vi "setSpectTempSetpoint.vi"(8 "error in (no error)":errorcluster, 9 "command_setSpectTempSetpoint":T1, 10 "model in":refnum<class "IModel.lvclass">, 11 "EnabledState in":refnum<class "EnabledState.lvclass">) -> (0 "error out":errorcluster, 2 "model out":refnum<class "IModel.lvclass">, 3 "EnabledState out":refnum<class "EnabledState.lvclass">)   [LabVIEW 2016, in "States.lvlib" / "EnabledState.lvclass"]
uses:
  EnabledState.lvclass
  IModel/IModel.lvclass
  ts_sallv_sedspectrometer/DataTypes/command_setSpectTempSetpoint.ctl
  DefaultState/DefaultState.lvclass
  ts_sallv_sedspectrometer/SALLV_sedSpectrometer.lvlib
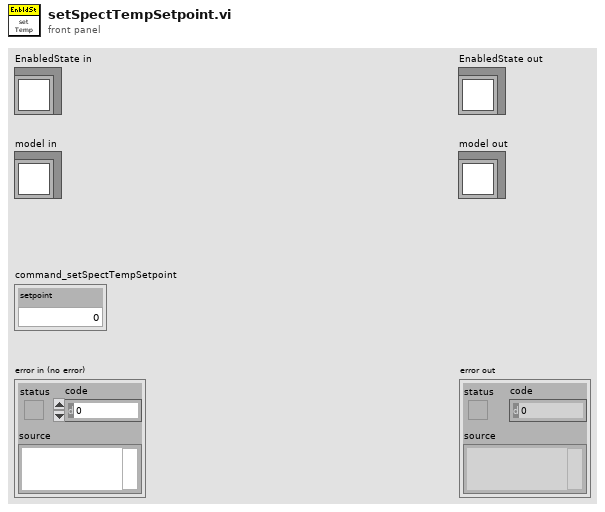
[diagram p1: front panel]
types:
  T1 = typedef "SALLV_sedSpectrometer.lvlib/command_setSpectTempSetpoint.ctl" = cluster{"setpoint":sgl}
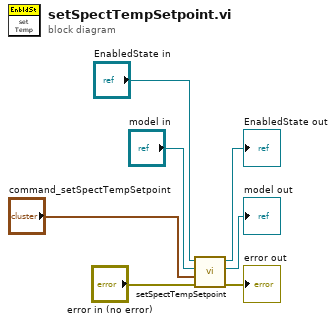
[diagram p0: block diagram]
diagram:
  n1 = call-parent "setSpectTempSetpoint.vi"("error in (no error)"="error in (no error)", "command_setSpectTempSetpoint"="command_setSpectTempSetpoint", "model in"="model in", "DefaultState in"="EnabledState in") -> ("error out"=→"error out":errorcluster, "model out"=→"model out":refnum<class "IModel.lvclass">, "DefaultState out"=→"EnabledState out":refnum<class "EnabledState.lvclass">)  [unwired: 5 in]
